vi "Method_Const.vi"(5 "Input A":refnum<class "Abs_Single Float.lvclass">) -> (1 "Result":T1)   [LabVIEW 2021, in "Add_SGL.lvclass"]
uses:
  Add_SGL.lvclass
  Abs_Types/Single Float/Abs_Single Float.lvclass
  C:/Program Files (x86)/National Instruments/LabVIEW 2021/vi.lib/TSA/Abstract Data Classes/Abs_Types/Numeric/Abs_Numeric.lvclass
  Abs_Type.ctl
  C:/TSA/LV_Abstract/Source/Functions/Support/Function/Two Terminal/SGL/AbsFunc_Two Term_SGL.lvclass
  C:/Program Files (x86)/National Instruments/LabVIEW 2021/vi.lib/TSA/Abstract Data Classes/Abs_Types/Single Float/Abs_Single Float.lvclass
  Support/Function/Two Terminal/SGL/AbsFunc_Two Term_SGL.lvclass/AbsFunc_Two Term_SGL.ctl
  Support/Function/Two Terminal/SGL/Properties/Write Numeric A.vi
  Support/Function/Two Terminal/SGL/Properties/Write Numeric B.vi
  Constants/Support/SGL/Const_SGL.lvclass
panel:
  in  "Value":sgl
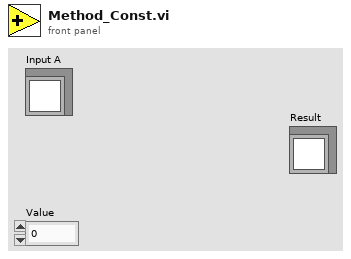
[diagram p1: front panel]
types:
  T1 = typedef "Add_SGL.lvclass/Abs_Type.ctl" = refnum<class "Abs_Single Float.lvclass">
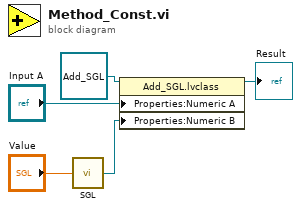
[diagram p0: block diagram]
diagram:
  n1 = call "SGL.vi"("Value"="Value") -> ("Constant"=w2:refnum<class "Abs_Single Float.lvclass">)  [unwired: 4 in]
  n2 = property class="Add_SGL.lvclass"(reference=refnum<class "Add_SGL.lvclass"> refnum ("Functions.lvlib:Numeric.lvlib:Add_SGL.lvclass"), "Properties:Numeric A"="Input A", "Properties:Numeric B"=w2) -> (reference out=→"Result":refnum<class "Add_SGL.lvclass">)  [unwired: 1 in, 1 out]
